vi "Handle getAll.vi"(8 "error in (no error)":errorcluster, 11 "Example Instrument in":refnum<class "Instrument.LN2.lvclass">) -> (0 "error out":errorcluster, 2 "getAll":variant, 3 "Example Instrument out":refnum<class "Instrument.LN2.lvclass">)   [LabVIEW 2019, in "Instrument.LN2.lvclass"]
uses:
  Instrument.LN2.lvclass
  Typedefs/Instrument.LN2.getAll--Cluster.ctl
  Instrument.LN2.lvclass/Instrument.LN2.ctl
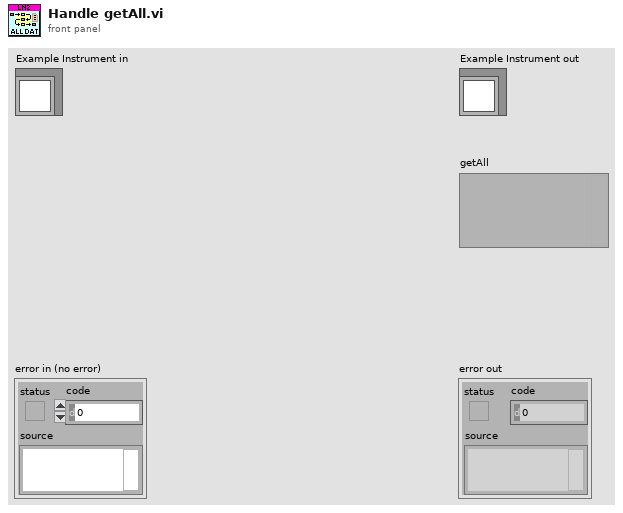
[diagram p1: front panel]
types:
  T1 = typedef "Instrument.LN2.lvclass/Instrument.LN2.getAll--Cluster.ctl" = cluster{"Net Weight(lbs)":dbl, "Gross Weight(lbs) ":dbl, "Tare Weight(lbs) ":dbl, "Empty":dbl}
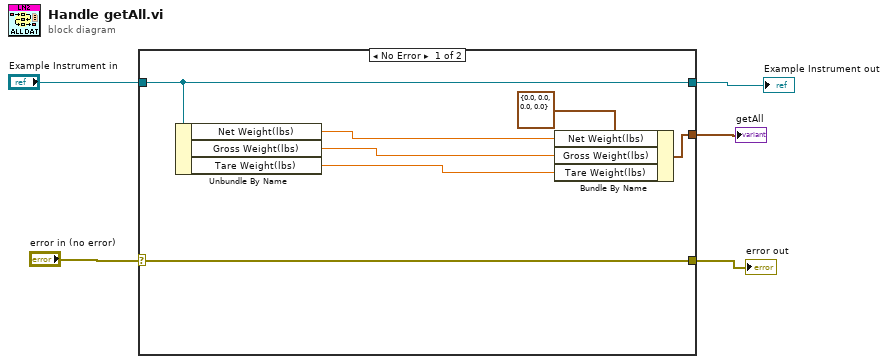
[diagram p0: block diagram]
diagram:
  n1 = case shown="No Error" "error in (no error)" {
    selector: "error in (no error)" -> [w8 w14]
    tunnel: "Example Instrument in" -> [w7 w13]
    tunnel: [w7 w13] -> w3
    tunnel: [w8 w14] -> w2
    tunnel: [w11 _] -> w1
    frame No Error {
      n2 = Unbundle By Name(w7) -> ("Net Weight(lbs)"=w6:dbl, "Gross Weight(lbs)"=w10:dbl, "Tare Weight(lbs)"=w9:dbl)
      n3 = Bundle By Name(cluster=T1 {"Net Weight(lbs)"=0.0, "Gross Weight(lbs) "=0.0, "Tare Weight(lbs) "=0.0, "Empty"=0.0} ("getAll"), "Net Weight(lbs)"=w6, "Gross Weight(lbs)"=w10, "Tare Weight(lbs)"=w9) -> (w11:T1)
    }
    frame Error {
    }
  }
  "error out" <- w2
  "Example Instrument out" <- w3
  "getAll" <- w1
